vi "Prefilter.Low Pass.vi"(8 "error in (no error)":errorcluster, 11 "Instrument.DAQ":refnum<class "Instrument.DAQ.lvclass">) -> (0 "error out":errorcluster, 3 "Instrument.DAQ out":refnum<class "Instrument.DAQ.lvclass">)   [LabVIEW 2019, in "Instrument.Lockin.lvlib" / "Instrument.DAQ.lvclass"]
uses:
  Instrument.DAQ.lvclass
  Instrument.DAQ.lvclass/Instrument.DAQ.ctl
  <vilib>/addons/Digital Filter Design/Process.llb/DFD Filtering (Wfm NChan).vi
  <vilib>/addons/Digital Filter Design/NI_DigFilterLicensed.lvlib
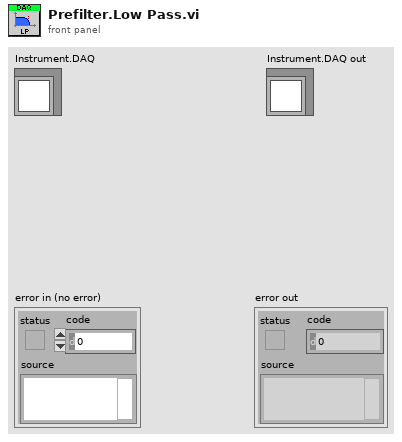
[diagram p1: front panel]
types:
  T1 = typedef "NI_DigFilterLicensed.lvlib/DFD Filter Obj.ctl" = cluster{"mSRate_Fs":dbl, "mSRate_Version":string, "mSRate_Comments":string, "mSRate_OrgCoef":T2, "mSRate_CurCoef":T2, "mSRate_Quantized?":bool, "mSRate_QCoef":T2, "mSRate_QSettings":T4[], "mSRate_Order":i32, "mSRate_Scaling":cluster{"mSRate_ScaleByPowerOf2?":bool, "mSRate_ScaleType":T6}}
  T2 = typedef "NI_DigFilterLicensed.lvlib/DFD Filter Coef.ctl" = cluster{"type":T3, "gain":dbl, "coef a (k)":dbl[], "coef b (v)":dbl[]}
  T3 = typedef "NI_DigFilterLicensed.lvlib/DFD Filter Structure Type Selector.ctl" = enum16{"Undefined", "FIR Direct Form", "FIR Direct Form Transposed", "FIR Symmetric", "FIR Antisymmetric", "IIR Direct Form I", "IIR Direct Form I Transposed", "IIR Direct Form II", "IIR Direct Form II Transposed", "IIR Cascaded Second Order Sections Form I", "IIR Cascaded Second Order Sections Form I Transposed", "IIR Cascaded Second Order Sections Form II", "IIR Cascaded Second Order Sections Form II Transposed", "Lattice Allpass (basic sections)", "Lattice Allpass (one multiplier sections)", "Lattice Allpass (normalized sections)", "Lattice AR (basic sections)", "Lattice AR (one multiplier sections)", "Lattice AR (normalized sections)", "Lattice MA (minimum phase)", "Lattice MA (maximum phase)", "Lattice ARMA (basic sections)", "Lattice ARMA (one multiplier sections)", "Lattice ARMA (normalized sections)"}
  T4 = typedef "NI_DigFilterLicensed.lvlib/dfd_Internal Quantization Settings.ctl" = cluster{"source":T5, "wl":i16, "iwl":i16, "overflow mode":enum16{"Saturation", "Wrap"}, "rounding mode":enum16{"Nearest", "Truncation"}, "signed?":bool}
  T5 = typedef "NI_DigFilterLicensed.lvlib/dfd_Internal Quantization Srcs.ctl" = u16
  T6 = typedef "NI_DigFilterLicensed.lvlib/DFD Coef Norm Type.ctl" = enum16{"No Norm", "Time Domain 1-Norm", "Time Domain 2-Norm", "Time Domain Inf-Norm"}
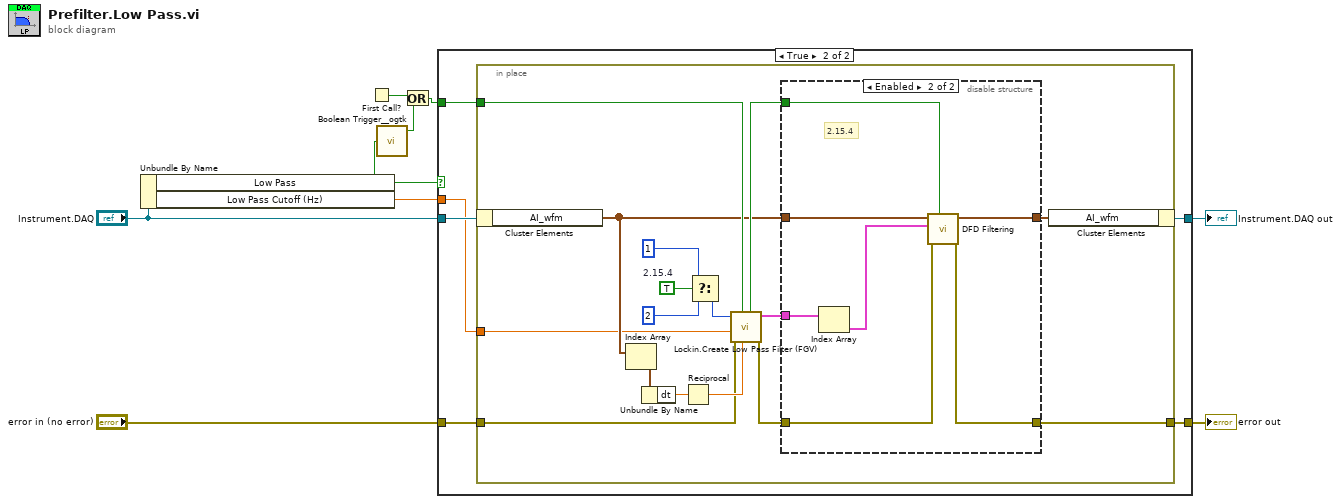
[diagram p0: block diagram]
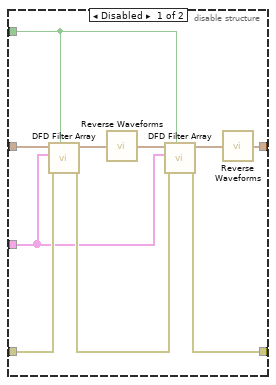
[diagram p3: hidden frame]
diagram:
  n1 = Unbundle By Name("Instrument.DAQ") -> ("Low Pass"=w3:bool, "Low Pass Cutoff (Hz)"=w1:dbl)
  n2 = First Call?() -> (First Call?: T/F=w5:bool)
  n3 = call <userlib>:"Boolean Trigger__ogtk.vi"("Boolean Input"=w3) -> ("Rising Edge"=w4:bool)  [unwired: 1 in, 1 out]
  n4 = Or(x=w5, y=w4) -> (x .or. y?=w2:bool)
  n5 = case shown="True" w3 {
    tunnel: "error in (no error)" -> [w10 w15]
    tunnel: [w10 w17] -> w8
    tunnel: "Instrument.DAQ" -> [w11 w14]
    tunnel: [w11 w13] -> w7
    tunnel: w2 -> [_ w16]
    tunnel: w1 -> [_ w12]
    frame False {
    }
    frame True {
      n6 = in-place {
        in-place-border: [w31] -> w17
        in-place-border: w16 -> [w30]
        in-place-border: w15 -> [w28]
        in-place-border: w12 -> [w23]
        w21 = TRUE  # 2.15.4
        n7 = in-place-cluster #1(w14) -> ("AI_wfm"=w24:waveform(dbl)[])
        n8 = Index Array(array=w24) -> (element=w32:waveform(dbl))  [unwired: 1 in]
        n9 = Unbundle By Name(w32) -> ("dt"=w33:dbl)
        n10 = Reciprocal(x=w33) -> (1/x=w29:dbl)
        n11 = Select(t=1 ("order"), s=w21, f=2 ("order")) -> (s? t:f=w20:i32)
        n12 = call "Lockin.Create Low Pass Filter (FGV).vi"("fs (Hz)"=w29, "init [F]"=w30, "error in (no error)"=w28, "Low Pass Cutoff (Hz)"=w23, "order"=w20) -> ("error out"=w27:errorcluster, "Filters out"=w22:T1[], "init out"=w26:bool)  [unwired: 4 in]
        n13 = disable-structure shown="Enabled" {
          disable-tunnel: [w39 w46] -> w31
          disable-tunnel: w27 -> [w38 w47]
          disable-tunnel: w26 -> [w37 w48]
          disable-tunnel: [w36 w49] -> w25
          disable-tunnel: w24 -> [w35 w50]
          disable-tunnel: w22 -> [w34 w45]
          frame Disabled {
            n14 = call "DFD Filter Array.vi"("init (F)"=w37, "error in (no error)"=w38, "filters"=w34, "signal in"=w35) -> ("error out"=w40:errorcluster, "signal out"=w41:waveform(dbl)[])  [unwired: 6 in]
            n15 = call "Reverse Waveforms.vi"("signal in"=w41) -> ("Array"=w43:waveform(dbl)[])
            n16 = call "DFD Filter Array.vi"("init (F)"=w37, "error in (no error)"=w40, "filters"=w34, "signal in"=w43) -> ("error out"=w39:errorcluster, "signal out"=w42:waveform(dbl)[])  [unwired: 6 in]
            n17 = call "Reverse Waveforms.vi"("signal in"=w42) -> ("Array"=w36:waveform(dbl)[])
          }
          frame Enabled {
            # "2.15.4"
            n18 = Index Array(array=w45) -> (element=w44:T1)  [unwired: 1 in]
            n19 = call-poly <vilib>:"DFD Filtering.vi"("init? (F)"=w48, "error in (no error)"=w47, "filter"=w44, "signal in"=w50) -> ("error out"=w46:errorcluster, "signal out"=w49:waveform(dbl)[])  [unwired: 6 in]
          }
        }
        n20 = in-place-cluster #1("AI_wfm"=w25) -> (w13:refnum<class "Instrument.DAQ.lvclass">)
      }
    }
  }
  "error out" <- w8
  "Instrument.DAQ out" <- w7
